vi "Perform Action.vi"(8 "error in (no error)":errorcluster, 10 "Input":variant, 11 "DIO DAQmx Fixed Freq PWM CFG in":refnum<class "DIO DAQmx Fixed Freq PWM CFG.lvclass">) -> (0 "error out":errorcluster, 2 "Output":variant, 3 "DIO DAQmx Fixed Freq PWM CFG out":refnum<class "DIO DAQmx Fixed Freq PWM CFG.lvclass">)   [LabVIEW 2023, in "DIO DAQmx Fixed Freq PWM CFG.lvclass"]
uses:
  DIO DAQmx Fixed Freq PWM CFG.lvclass
  D:/git/HAL/HAL GOOP4/DAQmx/DAQmx Base CFG/DAQmx Base CFG.lvclass
  DAQmx/DAQmx Base CFG/DAQmx Base CFG.lvclass/DAQmx Base CFG.ctl
  <resource>/objmgr/daqmx.rc
  DAQmx/DAQmx Base CFG/DAQmx Base CFG.lvclass
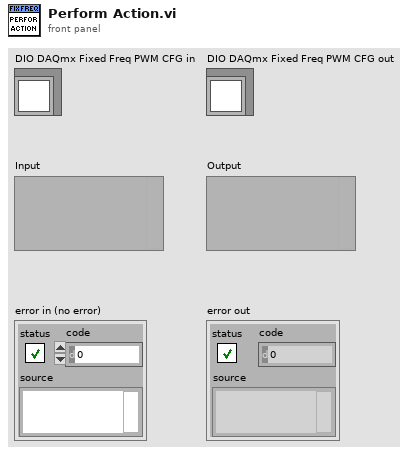
[diagram p1: front panel]
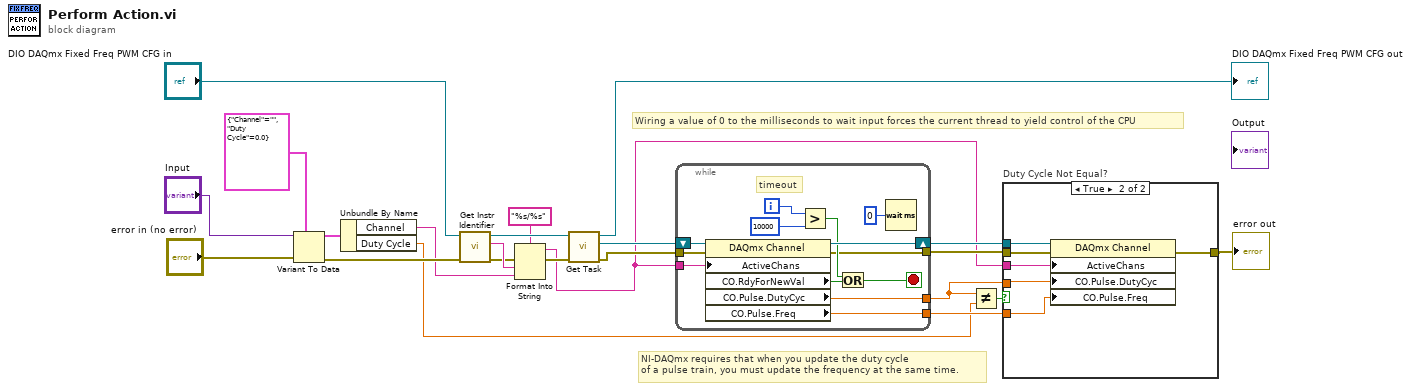
[diagram p0: block diagram]
diagram:
  # "Wiring a value of 0 to the milliseconds to wait input forces the current thread to yield control of the CPU"
  # "NI-DAQmx requires that when you update the duty cycle\nof a pulse train, you must update the frequency at the same time."
  n1 = Variant To Data(error in="error in (no error)", type=cluster{"Channel":string, "Duty Cycle":dbl} {"Channel"="", "Duty Cycle"=0.0}, Variant="Input") -> (data=w21:cluster{"Channel":string, "Duty Cycle":dbl}, error out=w22:errorcluster)
  n2 = Unbundle By Name(w21) -> ("Channel"=w17:string, "Duty Cycle"=w7:dbl)
  n3 = call-dynamic "Get Instr Identifier.vi"("error in (no error)"=w22, "Configuration Base in"="DIO DAQmx Fixed Freq PWM CFG in") -> ("error out"=w16:errorcluster, "Instr Identifier"=w18:string, "Configuration Base out"=w20:refnum<class "DIO DAQmx Fixed Freq PWM CFG.lvclass">)  [unwired: 7 in]
  n4 = Format Into String(format string="%s/%s", error in=w16, w18, w17) -> (resulting string=w9:string, error out=w15:errorcluster)  [unwired: 1 in]
  n5 = call "Get Task.vi"("error in (no error)"=w15, "DAQmx Base CFG in"=w20) -> ("error out"=w12:errorcluster, "Task"=w11:refnum<k21>, "DAQmx Base CFG out"=→"DIO DAQmx Fixed Freq PWM CFG out":refnum<class "DIO DAQmx Fixed Freq PWM CFG.lvclass">)  [unwired: 7 in]
  n6 = while {
    tunnel: [w35] -> w6
    tunnel: w12 -> [w34]
    tunnel: [w32] -> w8
    tunnel: w9 -> [w31]
    shift-right: [w36] -> w14
    shift-left: w11 -> [w33]
    tunnel: [w24] -> w10
    i -> [w29]
    stop <- w27 stop-if-true
    # "timeout"
    n7 = property class="DAQmx Channel"(reference=w33, error in=w34, "ActiveChans"=w31) -> (reference out=w36:refnum<k21>, error out=w24:errorcluster, "CO.RdyForNewVal"=w30:bool, "CO.Pulse.DutyCyc"=w35:dbl, "CO.Pulse.Freq"=w32:dbl)
    n8 = Greater?(x=w29, y=10000) -> (0:w26:bool)
    n9 = Or(x=w26, y=w30) -> (x .or. y?=w27:bool)
    n10 = Wait (ms)(milliseconds to wait=u32 0) -> ()  [unwired: 1 out]
  }
  n11 = Not Equal?(x=w6, y=w7) -> (x != y?=w13:bool)
  n12 = case "Duty Cycle Not Equal?" shown="True" w13 {
    tunnel: [w37 w43] -> w2
    tunnel: w10 -> [w37 w42]
    tunnel: w14 -> [_ w41]
    tunnel: w9 -> [_ w40]
    tunnel: w8 -> [_ w39]
    tunnel: w6 -> [_ w38]
    frame False {
    }
    frame True {
      n13 = property class="DAQmx Channel"(reference=w41, error in=w42, "ActiveChans"=w40, "CO.Pulse.DutyCyc"=w38, "CO.Pulse.Freq"=w39) -> (error out=w43:errorcluster)  [unwired: 1 out]
    }
  }
  "error out" <- w2
